vi "Do.vi"(8 "error in (no error)":errorcluster, 10 "Actor in":refnum<class "Actor.lvclass">, 11 "Addition Result Msg":refnum<class "Addition Result Msg.lvclass">) -> (0 "error out":errorcluster, 2 "Actor out":refnum<class "Actor.lvclass">)   [LabVIEW 2014, in "Addition Result Msg.lvclass"]
doc: "(<B>Filename</B>: Actor Framework.lvlib:Message.lvclass:Do.vi)\n\nDefines what a message does when it is received by an actor. Generally, a message instructs an actor to invoke one of its methods. By default, this method does nothing. A child class must override it to define behavior. Create a child class by using the Actor Framework Message Maker dialog box."
uses:
  Addition Result Msg.lvclass
  <vilib>/ActorFramework/Actor/Actor.lvclass
  Calculator Actor Class/Calculator Actor.lvclass
  Addition Result Msg.lvclass/Addition Result Msg.ctl
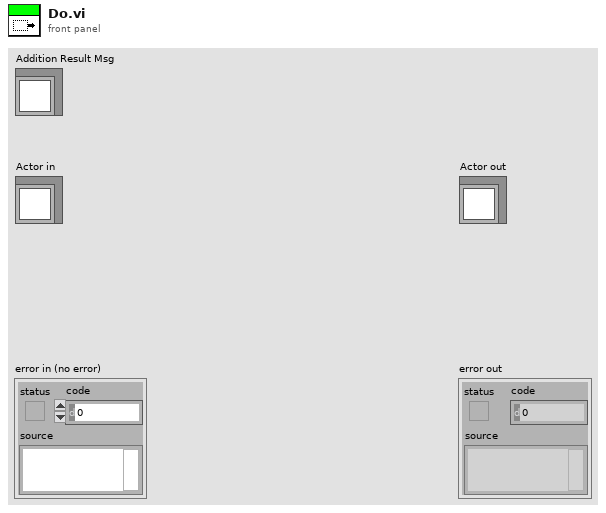
[diagram p1: front panel]
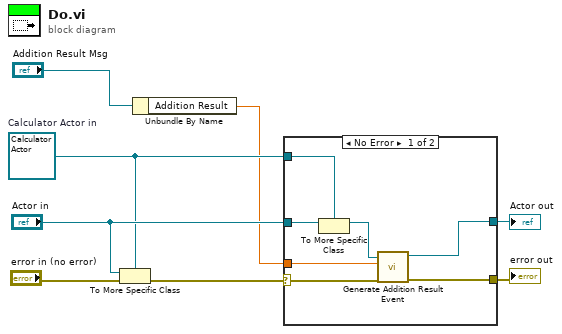
[diagram p0: block diagram]
diagram:
  w3 = refnum<class "Calculator Actor.lvclass"> refnum  # Calculator Actor in
  n1 = To More Specific Class(target class=w3, reference="Actor in", error in="error in (no error)") -> (error out=w7:errorcluster)  [unwired: 1 out]
  n2 = Unbundle By Name("Addition Result Msg") -> ("Addition Result"=w1:dbl)
  n3 = case shown="No Error" w7 {
    selector: w7 -> [w14 w16]
    tunnel: "Actor in" -> [w15 w17]
    tunnel: w3 -> [w13 _]
    tunnel: [w11 w16] -> w5
    tunnel: [w10 w17] -> w4
    tunnel: w1 -> [w9 _]
    frame No Error {
      n4 = To More Specific Class(target class=w13, reference=w15) -> (specific class reference=w12:refnum<class "Calculator Actor.lvclass">)  [unwired: 1 in, 1 out]
      n5 = call "Generate Addition Result Event.vi"("error in (no error)"=w14, "Addition Result"=w9, "Calculator Actor in"=w12) -> ("error out"=w11:errorcluster, "Calculator Actor out"=w10:refnum<class "Calculator Actor.lvclass">)  [unwired: 7 in]
    }
    frame Error {
    }
  }
  "error out" <- w5
  "Actor out" <- w4
